vi "Initialize Group Local Data.vi"(8 "error in (no error)":errorcluster, 10 "Transfer Group":refnum<class "Transfer Group.lvclass">, 11 "UDP Transceiver in":refnum<class "DSF UDP Transceiver.lvclass">) -> (0 "error out":errorcluster, 1 "group data":string, 3 "UDP Transceiver out":refnum<class "DSF UDP Transceiver.lvclass">)   [LabVIEW 2017, in "DSF Core.lvlib" / "DSF UDP Transceiver.lvclass"]
uses:
  DSF UDP Transceiver.lvclass
  Classes/Transfer Group/Transfer Group.lvclass
  DSF UDP Transceiver.lvclass/DSF UDP Transceiver.ctl
  Classes/Buffer/Buffer.lvclass
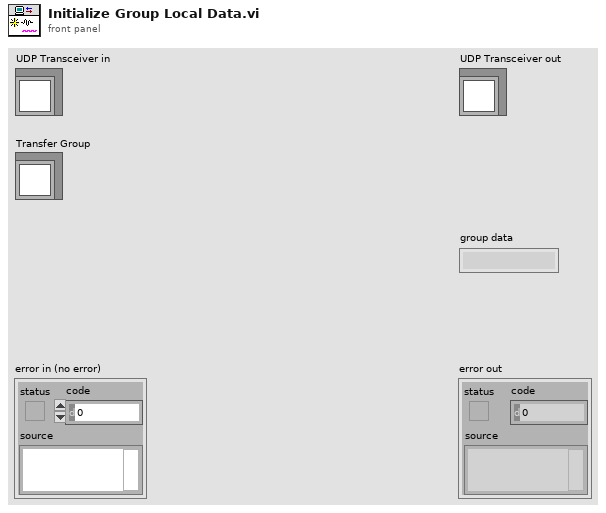
[diagram p1: front panel]
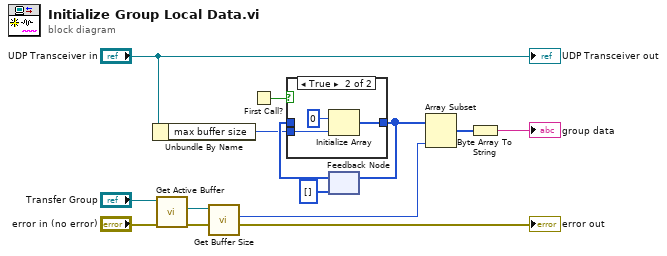
[diagram p0: block diagram]
diagram:
  n1 = Unbundle By Name("UDP Transceiver in") -> ("max buffer size"=w5:u64)
  n2 = call "Get Active Buffer.vi"("error in (no error)"="error in (no error)", "Transfer Group in"="Transfer Group") -> ("error out"=→"error out":errorcluster, "Buffer"=w11:refnum<class "Buffer.lvclass">)  [unwired: 7 in, 1 out]
  n3 = call "Get Buffer Size.vi"("Buffer in"=w11) -> ("buffer size"=w3:u64)  [unwired: 9 in, 1 out]
  n4 = First Call?() -> (First Call?: T/F=w8:bool)
  n5 = feedback #1(u8[] []) -> (w6:u8[])
  n6 = case shown="True" w8 {
    tunnel: w5 -> [_ w17]
    tunnel: [w14 w15] -> w4
    tunnel: w6 -> [w14 _]
    frame False {
    }
    frame True {
      n7 = Initialize Array(u8 0 ("element"), w17) -> (w15:u8[])
    }
  }
  n8 = feedback-in #1(w4) -> ()
  n9 = Array Subset(array=w4, length=w3) -> (w2:u8[])  [unwired: 1 in]
  n10 = Byte Array To String(unsigned byte array=w2) -> (string=→"group data":string)
  "UDP Transceiver out" <- "UDP Transceiver in"
